vi "Motor_Excel_to_Array(OK).vi"() -> ()   [LabVIEW 2016]
uses:
  <vilib>/addons/_office/excel.llb/Excel Get Data ([dbl]).vi
  <vilib>/Utility/NIReport.llb/NI_report.lvclass
  <vilib>/Utility/NIReport.llb/Excel/NI_Excel.lvclass
  <vilib>/addons/_office/NI_ReportGenerationToolkit.lvlib
  <vilib>/gmath/NI_Gmath.lvlib
panel:
  in  "Path":path=path "C:/Users/YENPEI/Desktop/LabView/20.2_Motor_Performace - accel/Peak.xls"
  in  "Tab Control":T1(tab)
  out "XY Graph":cluster{"data":dbl[], "data":dbl[]}[](graph)
  out "Speed -MotorTorque - Curve":T2(graph)={"array type (2D Dbl)"=[0.0, 5.0, 10.0, 15.0, 20.0, 25.0, 30.0, 35.0, 40.0, 45.0, 50.0, 55.0, 60.0, 65.0, 70.0, 75.0, 80.0, 85.0, 90.0, 95.0, 100.0, 105.0, 110.0, 115.0, 120.0, 125.0, 130.0, 135.0, 140.0, 145.0, 150.0, 155.0, 160.0, 165.0, 170.0, 175.0, 180.0, 185.0, 190.0, 195.0, 200.0, 205.0, 210.0, 215.0, 220.0, 225.0, 230.0, 235.0, 240.0, 245.0], "array type (2D Dbl)"=[7.64, 4.95, 6.83, 9.7, 4.25, 5.21, 3.69, 9.63, 7.28, 4.87, 6.61, 3.48, 3.51, 5.43, 7.79, 2.74, 3.77, 9.97, 2.54, 5.19, 9.7, 5.12, 1.95, 1.46, 2.93, 2.02, 4.5, 5.86, 6.09, 5.11, 1.22, 8.82, 1.81, 7.21, 5.19, 4.2, 7.97, 6.75, 2.71, 3.86, 1.49, 3.44, 5.75, 5.05, 3.16, 8.68, 8.7, 4.07, 5.28, 3.4]}
  out "Motor Max Torque":T2(graph)={"array type (2D Dbl)"=[0.0, 5.0, 10.0, 15.0, 20.0, 25.0, 30.0, 35.0, 40.0, 45.0, 50.0, 55.0, 60.0, 65.0, 70.0, 75.0, 80.0, 85.0, 90.0, 95.0, 100.0, 105.0, 110.0, 115.0, 120.0, 125.0, 130.0, 135.0, 140.0, 145.0, 150.0, 155.0, 160.0, 165.0, 170.0, 175.0, 180.0, 185.0, 190.0, 195.0, 200.0, 205.0, 210.0, 215.0, 220.0, 225.0, 230.0, 235.0, 240.0, 245.0], "array type (2D Dbl)"=[7.64, 4.95, 6.83, 9.7, 4.25, 5.21, 3.69, 9.63, 7.28, 4.87, 6.61, 3.48, 3.51, 5.43, 7.79, 2.74, 3.77, 9.97, 2.54, 5.19, 9.7, 5.12, 1.95, 1.46, 2.93, 2.02, 4.5, 5.86, 6.09, 5.11, 1.22, 8.82, 1.81, 7.21, 5.19, 4.2, 7.97, 6.75, 2.71, 3.86, 1.49, 3.44, 5.75, 5.05, 3.16, 8.68, 8.7, 4.07, 5.28, 3.4]}
  out "Motor Power Curve":T2(graph)={"array type (2D Dbl)"=[0.0, 5.0, 10.0, 15.0, 20.0, 25.0, 30.0, 35.0, 40.0, 45.0, 50.0, 55.0, 60.0, 65.0, 70.0, 75.0, 80.0, 85.0, 90.0, 95.0, 100.0, 105.0, 110.0, 115.0, 120.0, 125.0, 130.0, 135.0, 140.0, 145.0, 150.0, 155.0, 160.0, 165.0, 170.0, 175.0, 180.0, 185.0, 190.0, 195.0, 200.0, 205.0, 210.0, 215.0, 220.0, 225.0, 230.0, 235.0, 240.0, 245.0], "array type (2D Dbl)"=[7.64, 4.95, 6.83, 9.7, 4.25, 5.21, 3.69, 9.63, 7.28, 4.87, 6.61, 3.48, 3.51, 5.43, 7.79, 2.74, 3.77, 9.97, 2.54, 5.19, 9.7, 5.12, 1.95, 1.46, 2.93, 2.02, 4.5, 5.86, 6.09, 5.11, 1.22, 8.82, 1.81, 7.21, 5.19, 4.2, 7.97, 6.75, 2.71, 3.86, 1.49, 3.44, 5.75, 5.05, 3.16, 8.68, 8.7, 4.07, 5.28, 3.4]}
  out "Speed - RoadTorque - Curve2":T2(graph)={"array type (2D Dbl)"=[0.0, 5.0, 10.0, 15.0, 20.0, 25.0, 30.0, 35.0, 40.0, 45.0, 50.0, 55.0, 60.0, 65.0, 70.0, 75.0, 80.0, 85.0, 90.0, 95.0, 100.0, 105.0, 110.0, 115.0, 120.0, 125.0, 130.0, 135.0, 140.0, 145.0, 150.0, 155.0, 160.0, 165.0, 170.0, 175.0, 180.0, 185.0, 190.0, 195.0, 200.0, 205.0, 210.0, 215.0, 220.0, 225.0, 230.0, 235.0, 240.0, 245.0], "array type (2D Dbl)"=[7.64, 4.95, 6.83, 9.7, 4.25, 5.21, 3.69, 9.63, 7.28, 4.87, 6.61, 3.48, 3.51, 5.43, 7.79, 2.74, 3.77, 9.97, 2.54, 5.19, 9.7, 5.12, 1.95, 1.46, 2.93, 2.02, 4.5, 5.86, 6.09, 5.11, 1.22, 8.82, 1.81, 7.21, 5.19, 4.2, 7.97, 6.75, 2.71, 3.86, 1.49, 3.44, 5.75, 5.05, 3.16, 8.68, 8.7, 4.07, 5.28, 3.4]}
  out "XY Graph 2":cluster{"data":dbl[], "data":dbl[]}[](graph)
  out "slope_value_(%) 2":dbl format="%.1f"
  out "Motor_Max_Torque(Nm) 2":dbl format="%.2f"
  out "Motor_Max_Power(kW)":dbl format="%.2f"
  out "Vehicle_speed_Hi(kph)@ Slope":dbl format="%.2f"
  out "Vehicle_speed_Lo(kph)@ Slope":dbl format="%.2f"
  out "Tire_Torque Array(kph_Nm)":dbl[][](array[numeric]) format="%#.1f"
  out "Motor_Torque_Orignal":dbl[][](array[numeric])
  in  "window state (normal)":T3(ring)=enum."normal"
  in  "report type":T4(ring)=enum."Excel"
  out "Vehicle_speed_(m/s)":dbl[](array[numeric])
  out "Vehicle_speed_(km/h)":dbl[](array[numeric])
  out "Road_Resistance_Array (kph_Nm)":dbl[][](array[numeric]) format="%#.1f"
  out "Road_Load 1 (Aero)":dbl[](array[numeric])
  out "Road_Load 2 (Roll)":dbl=0.7
  out "Road_Load_3(slope)":dbl=0.7
  out "New_Motor_Torque_Array (rpm_Nm)":dbl[][](array[numeric])
  in  "Road_Slope_(%)":sgl(slide) min=0 max=30 step=1 scale=0.0..30.0
  in  "Trie_HWRatio_(%)":dbl=75.0
  out "Front_Area(m^2)":dbl
  out "Tire_Radius(m)":dbl=0.3835
  in  "Mass_AddFactor_(-)":dbl=1.04
  in  "Tire_Diameter_ (in)":dbl=17.5
  in  "Tire_Height_(mm)":dbl=215.0
  out "Trie Skip coefficient(-)":dbl=0.03
  in  "Reducer_Ratio_(-)":dbl=5.13
  out "rolling friction_coefficient_(-)":dbl=0.01
  out "Airdensity(kg/m^3)":dbl=1.225
  out "Graviational_constant_(m/s^2)":dbl=9.81
  out "areo_dynamic_coefficient_(-)":dbl=0.7
  in  "Powertrain_eff_(%)":dbl=85.0
  in  "Vehicle_Load_(kg)":dbl=9900.0
  in  "Vehicle_width_(m)":dbl=2.3
  in  "Vehicle_Height_m)":dbl=3.0
  in  "Front_Area_constant(-)":dbl=1.0
  out "slope_value_(%)":dbl format="%.1f"
  in  "Table":bool=TRUE
  out "Max slope_angle_(deg)":dbl format="%.1f"
  out "Max slope_value_(%)":dbl format="%.1f"
  out "Vehicle_Max_speed_(kph)":dbl format="%.2f"
  in  "Torque _(Nm) @ Max_Motor_speed":dbl=500.0
  in  "Max_Motor_speed (rpm)":dbl=4000.0
  out "Vehicle_Max_speed":dbl format="%.2f"
  out "Road_Loading_Torque":dbl format="%.2f"
  out "Vehicle_Torque_Max_speed":dbl format="%.2f"
  out "Motor_Max_Torque(Nm)":dbl format="%.2f"
  in  "Motor _Max Torque (Nm)":dbl=2000.0
  in  "Motor_speed @ Max Torque (rpm)":dbl=1000.0
  out "Vehicle_spped_Array (m/s_Nm) 2":dbl[][](array[numeric])
  out "Vehicle_Total_Array":dbl[][](array[numeric]) format="%.2f"
  out "vehicle speed vs Distance":cluster{dbl[], dbl[]}(graph)
  out "Aceel time vs vehicle speed":cluster{dbl[], dbl[]}(graph)
  in  "Max Distance [m]":i32=400 min=0 max=400 step=1
  in  "Max Accel  time [sec]":i32=20 min=0 max=20 step=1
  in  "Max Items":i32=29 min=0 max=30 step=1
  in  "Stop Mode":i32 min=0 max=3 step=1
  in  "Max Vehicel Speed [kph]":i32=60 min=0 max=100 step=1
  out "Aceel time vs Distance":cluster{dbl[], dbl[]}(graph)
  out "Accel_Result":dbl[](array[numeric]) format="%.2f"
  # "Max Vehicle Speed\nBetween"
  # "~"
  # "最大爬坡度"
  # "極速(km/hr)"
  # "檢查馬達最大轉速 Nmax (rpm)     與扭力(Nm)"
  # "¦pªGTable data µL°¨¹F³Ì¤jÂà³t , Table¶s Disable¡A«h¤â°Ê¿é¤J¤U¤è"
  # "檢查馬達最大扭力(Nm)"
  # "¦pªGTable data µL°¨¹F³Ì¤j§á¤O ,  Table¶s Disable ¡A«h¤â°Ê¿é¤J¤U¤è"
  # "Finak \n車速 m/s"
  # "Motor\nrpm"
  # "Motor\nrpm"
  # "Tire Drive\nN"
  # "Aceel Drive\nN"
  # "Aceel \n1/sec"
  # "time  \nsec"
  # "車速 m/s"
  # "車速 kph"
  # "Drag"
  # "Roll"
  # "Drag+Roll"
  # "Distance\nm"
  # "Final \n車速 kph"
  # "Total Time\n[sec]"
  # "Total Distance\n[m]"
  # "Mode =0"
  # "Max =30"
  # "Item"
  # "Final \n車速 kph"
  # "Total Time\n[sec]"
  # "Total Distance\n[m]"
  # "Mode =1"
  # "Max =100"
  # "Mode =2"
  # "Max =15"
  # "Mode =3"
  # "Max =300"
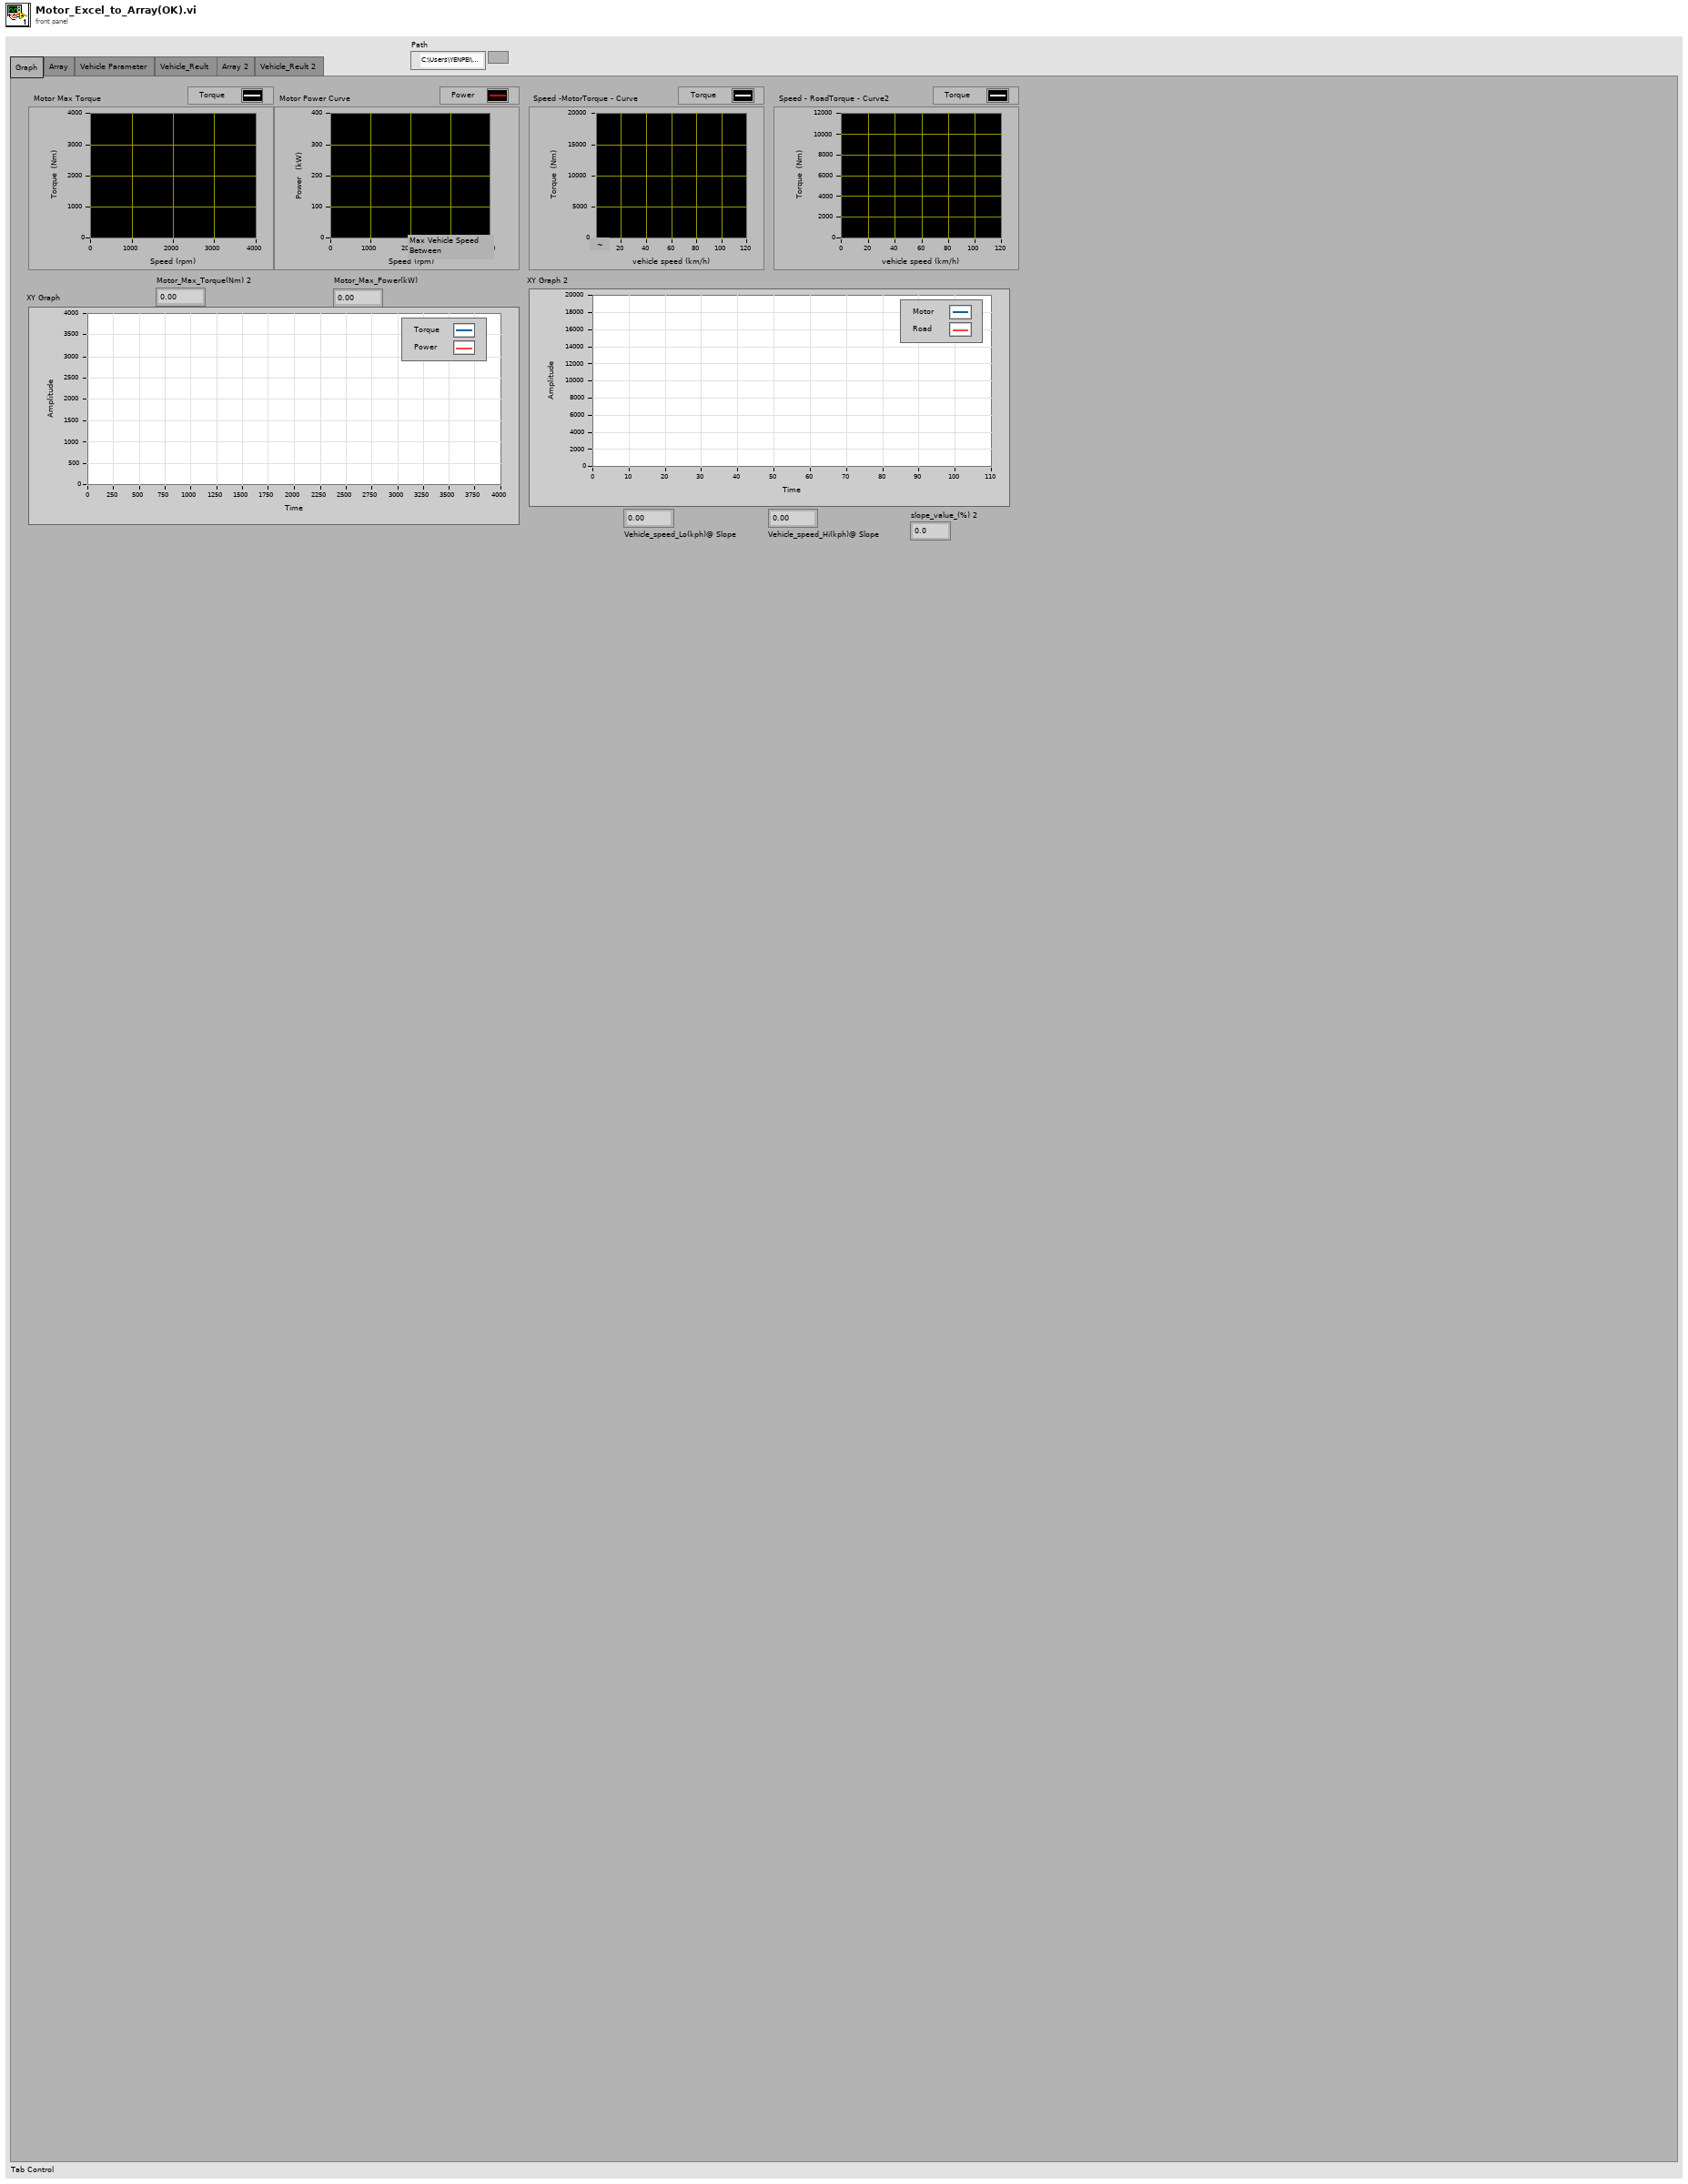
[diagram p1: front panel]
types:
  T1 = enum32{"Graph", "Array", "Vehicle Parameter", "Vehicle_Reult", "Array 2", "Vehicle_Reult 2"}
  T2 = cluster{"array type (2D Dbl)":dbl[], "array type (2D Dbl)":dbl[]}
  T3 = enum16{"maximized", "minimized", "normal", "no change"}
  T4 = enum16{"Standard Report", "HTML", "Word", "Excel"}
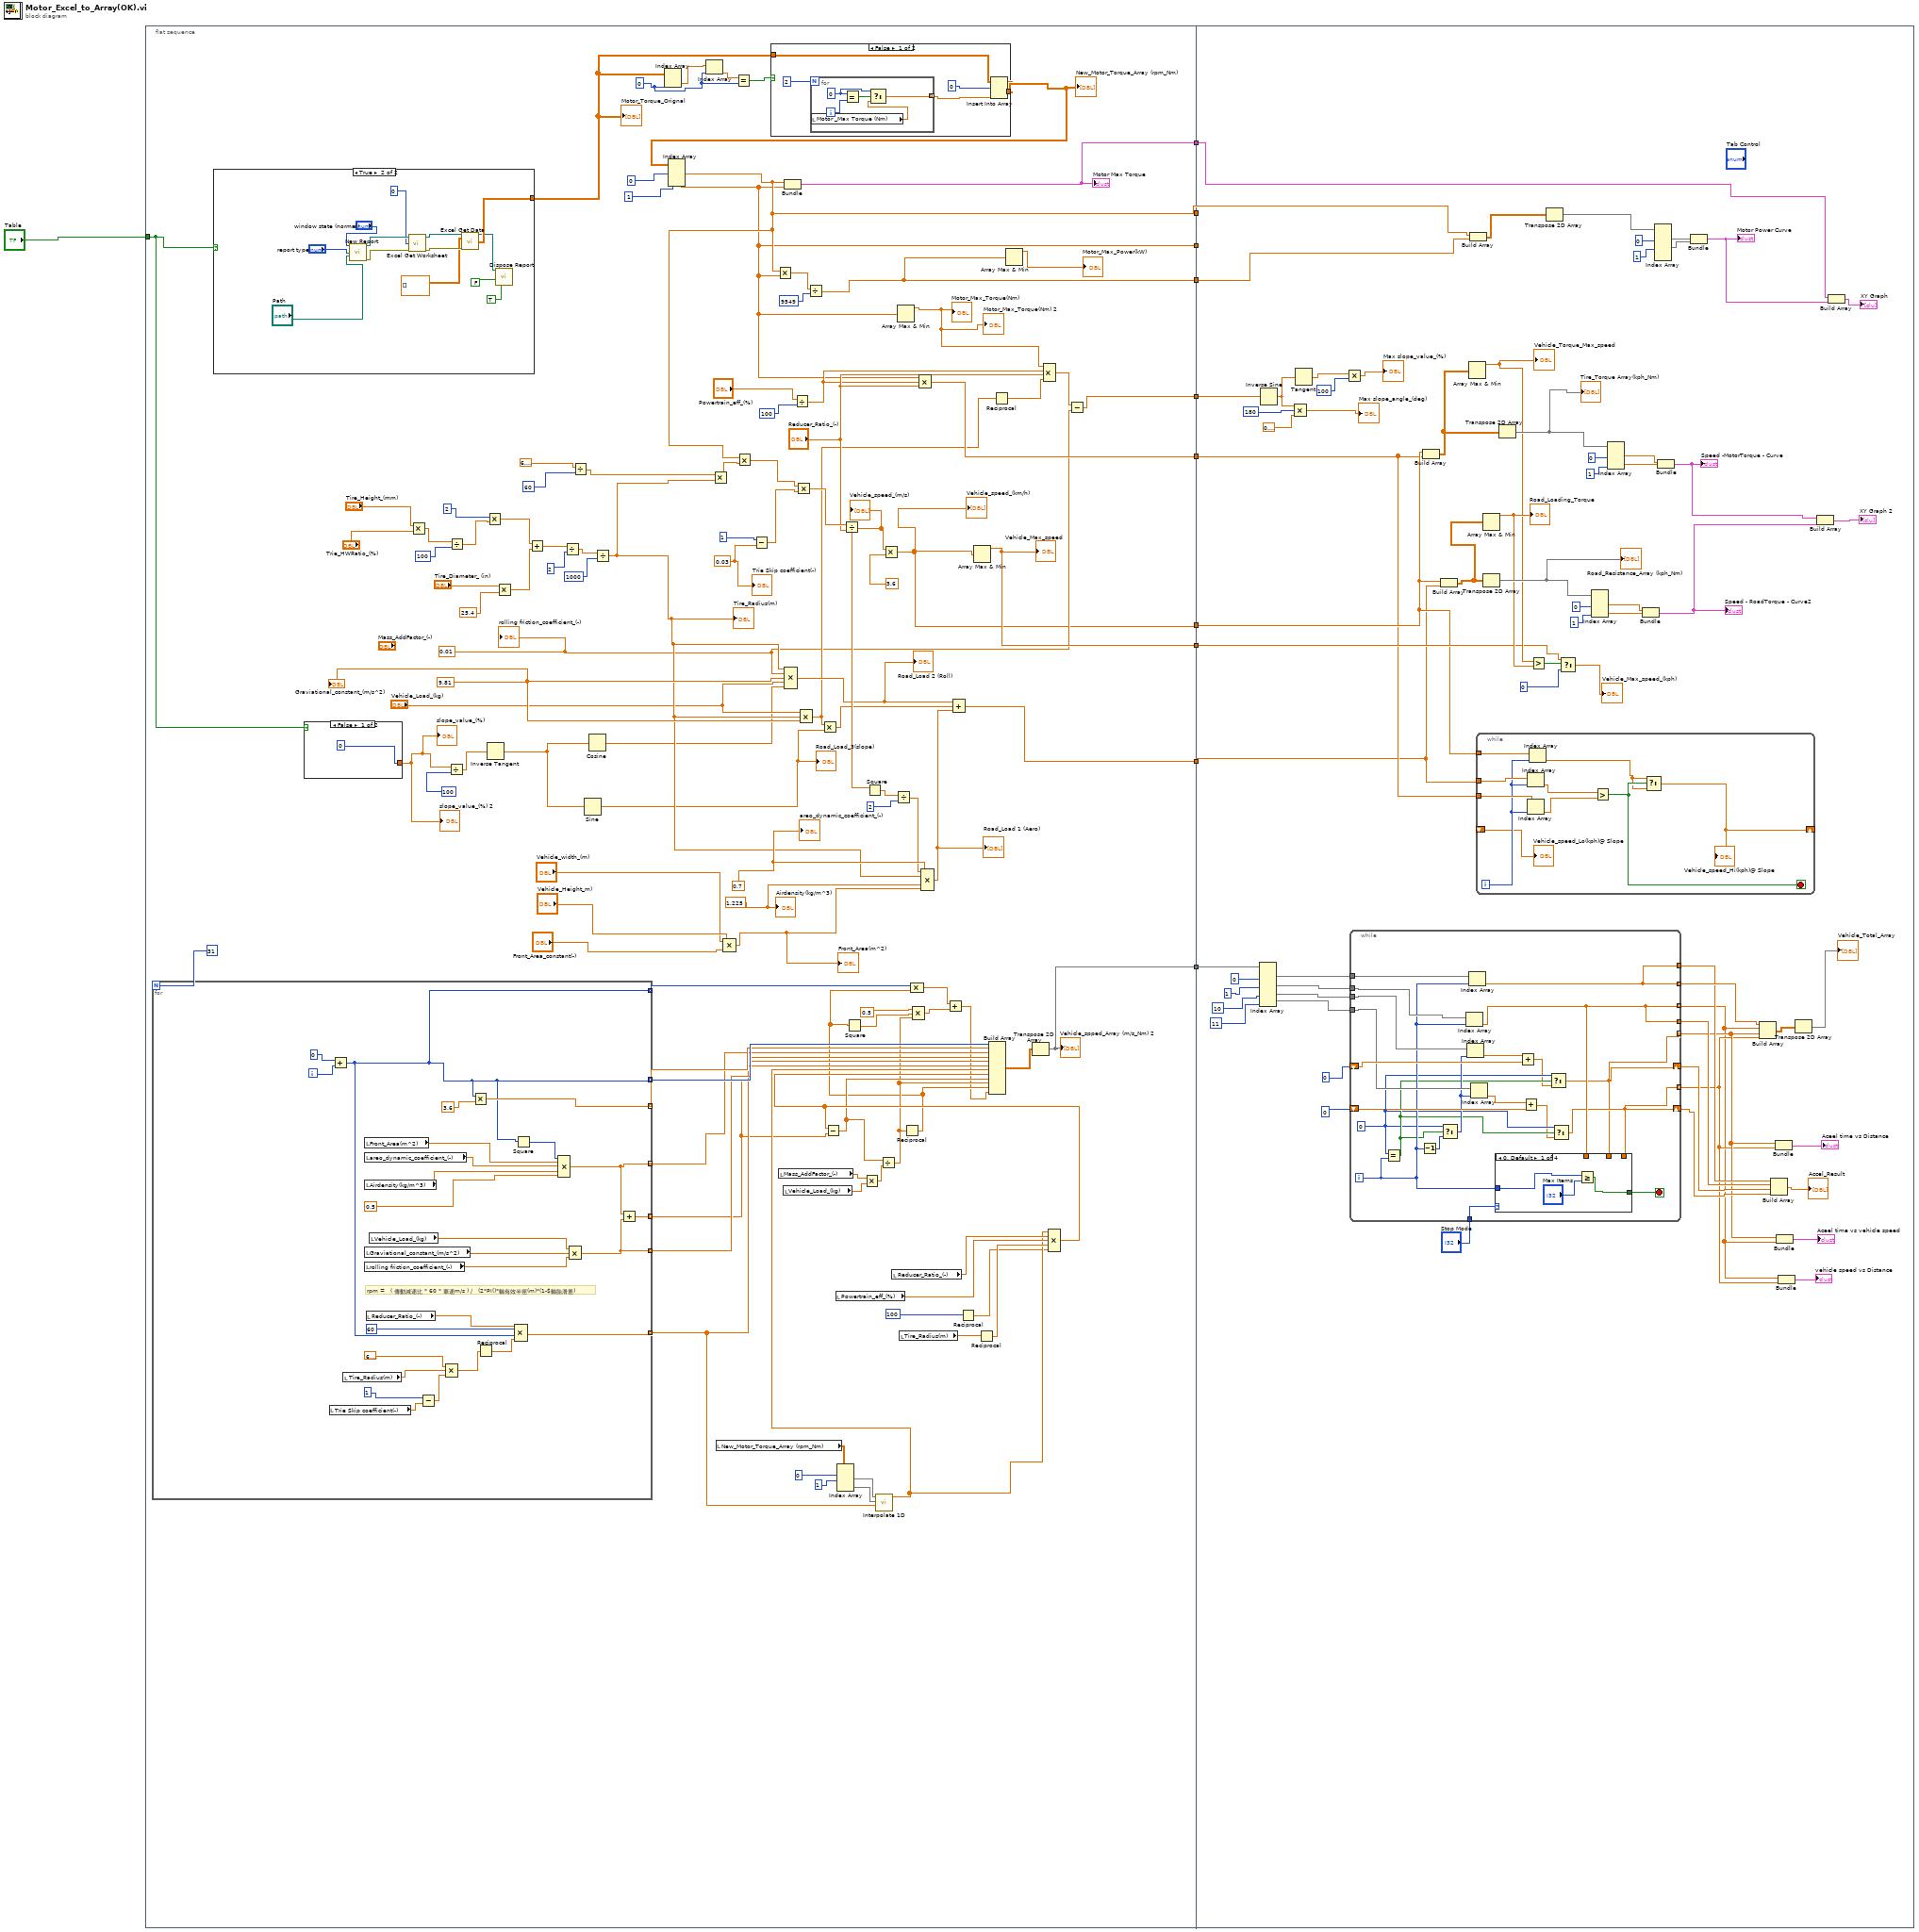
[diagram p0: block diagram]
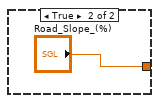
[diagram p3: hidden frame]
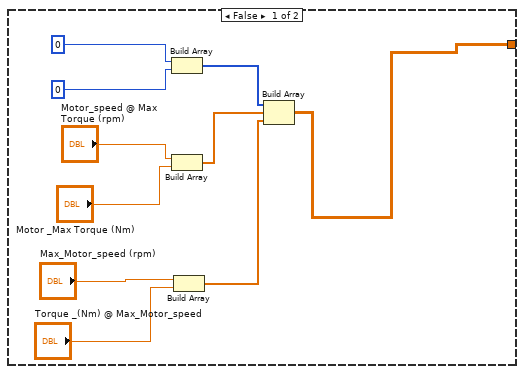
[diagram p4: hidden frame]
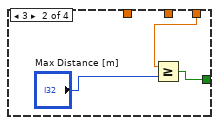
[diagram p5: hidden frame]
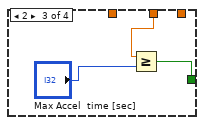
[diagram p6: hidden frame]
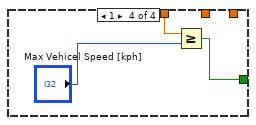
[diagram p7: hidden frame]
diagram:
  n1 = flat-sequence {
    tunnel: [w22] -> w10
    tunnel: [w15] -> w9
    tunnel: [w23] -> w8
    tunnel: [w60] -> w7
    tunnel: [w83] -> w6
    tunnel: [w82] -> w5
    tunnel: "Table" -> [w72]
    tunnel: [w71] -> w4
    tunnel: [w63] -> w3
    tunnel: [w59] -> w2
    tunnel: [w24] -> w1
    tunnel: w10 -> [_]
    tunnel: w9 -> [w245]
    tunnel: w8 -> [w246]
    tunnel: w7 -> [w186]
    tunnel: w6 -> [w185]
    tunnel: w5 -> [w184]
    tunnel: w4 -> [w227]
    tunnel: w3 -> [w219]
    tunnel: w2 -> [w218]
    tunnel: w1 -> [w212]
    frame #0 {
      w19 = 0
      w90 = 0.7
      w64 = 0.01
      w89 = 1.225
      w79 = 9.81
      w98 = 0.03
      n2 = for {
        N: 31 -> [_]
        tunnel: [w133] -> w56 mode=indexing
        tunnel: [w155] -> w55 mode=indexing
        tunnel: [w146] -> w54 mode=indexing
        tunnel: [w145] -> w53 mode=indexing
        tunnel: [w144] -> w38 mode=indexing
        tunnel: [w134] -> w48 mode=indexing
        tunnel: [w133] -> w33 mode=indexing
        i -> [w157]
        # "rpm =   ( 傳動減速比 * 60 * 車速m/s ) /   (2*PI()*輪有效半徑(m)*(1-$輪胎滑差)"
        n3 = local read "Trie Skip coefficient(-)"() -> (w137:dbl)
        n4 = Add(x=0, y=w157) -> (x+y=w133:i32)
        n5 = local read "Tire_Radius(m)"() -> (w135:dbl)
        n6 = local read "Front_Area(m^2)"() -> (w148:dbl)
        n7 = local read "areo_dynamic_coefficient_(-)"() -> (w149:dbl)
        n8 = local read "Airdensity(kg/m^3)"() -> (w150:dbl)
        n9 = local read "Graviational_constant_(m/s^2)"() -> (w152:dbl)
        n10 = local read "rolling friction_coefficient_(-)"() -> (w153:dbl)
        n11 = local read "Reducer_Ratio_(-)"() -> (w143:dbl)
        n12 = local read "Vehicle_Load_(kg)"() -> (w154:dbl)
        n13 = Subtract(x=1, y=w137) -> (x-y=w136:dbl)
        n14 = Compound Arithmetic op=MULTIPLY(6.283185307179586, w135, w136) -> (w140:dbl)
        n15 = Multiply(x=w133, y=3.6) -> (x*y=w155:dbl)
        n16 = Reciprocal(x=w140) -> (1/x=w141:dbl)
        n17 = Compound Arithmetic op=MULTIPLY(w143, 60, w133, w141) -> (w134:dbl)
        n18 = Square(x=w133) -> (x^2=w147:i32)
        n19 = Compound Arithmetic op=MULTIPLY(w147, w148, w149, w150, 0.5) -> (w146:dbl)
        n20 = Compound Arithmetic op=MULTIPLY(w154, w152, w153) -> (w145:dbl)
        n21 = Add(x=w146, y=w145) -> (x+y=w144:dbl)
      }
      n22 = case shown="True" w72 {
        tunnel: [w165 w177] -> w17
        frame False {
          n23 = Build Array(0, 0) -> (w166:i32[])
          n24 = Build Array("Motor_speed @ Max Torque (rpm)", "Motor _Max Torque (Nm)") -> (w161:dbl[])
          n25 = Build Array("Max_Motor_speed (rpm)", "Torque _(Nm) @ Max_Motor_speed") -> (w164:dbl[])
          n26 = Build Array(w166, w161, w164) -> (w165:dbl[][])
        }
        frame True {
          n27 = call <vilib>:"New Report.vi"("window state (normal)"="window state (normal)", "report type"="report type", "template (empty)"="Path") -> ("report out"=w182:refnum<class "NI_report.lvclass">, "error out"=w183:errorcluster)  [unwired: 11 in]
          n28 = call <vilib>:"Excel Get Worksheet.vi"("report in"=w182, "worksheet index (0)"=0, "error in (no error)"=w183) -> ("report out"=w181:refnum<class "NI_report.lvclass">, "error out"=w180:errorcluster)  [unwired: 11 in]
          n29 = call-poly <vilib>:"Excel Get Data.vi"("report in"=w181, "data type"=dbl[][] [], "error in (no error)"=w180) -> ("report out"=w173:refnum<class "NI_report.lvclass">, "data"=w177:dbl[][])  [unwired: 10 in, 1 out]
          n30 = call-dynamic "Dispose Report.vi"("report in"=w173, "save changes? (F)"=FALSE, "close report? (T)"=TRUE) -> ()  [unwired: 12 in, 1 out]
        }
      }
      "Motor_Torque_Orignal" <- w17
      n31 = case shown="False" w72 {
        tunnel: [0 "Road_Slope_(%)"] -> w12
        frame False {
        }
        frame True {
        }
      }
      "slope_value_(%)" <- w12
      "slope_value_(%) 2" <- w12
      n32 = Multiply(x="Tire_Height_(mm)", y="Trie_HWRatio_(%)") -> (x*y=w112:dbl)
      n33 = Divide(x=w12, y=100) -> (x/y=w75:sgl)
      n34 = Divide(x=w112, y=100) -> (x/y=w107:dbl)
      n35 = Multiply(x=2, y=w107) -> (x*y=w106:dbl)
      n36 = Inverse Tangent(1:w75) -> (0:w76:sgl)
      n37 = Multiply(x="Tire_Diameter_ (in)", y=25.4) -> (x*y=w105:dbl)
      n38 = Add(x=w106, y=w105) -> (x+y=w102:dbl)
      n39 = Divide(x=w102, y=2) -> (x/y=w100:dbl)
      n40 = Divide(x=6.283185307179586, y=60) -> (x/y=w115:dbl)
      n41 = Sine(x=w76) -> (sin(x)=w58:sgl)
      "Road_Load_3(slope)" <- w58
      n42 = Cosine(x=w76) -> (cos(x)=w68:sgl)
      n43 = Divide(x=w100, y=1000) -> (x/y=w77:dbl)
      "Tire_Radius(m)" <- w77
      n44 = Index Array(array=w17, index (row)=w19) -> (element=w21:dbl[])  [unwired: 1 in]
      n45 = Index Array(array=w21, index=w19) -> (element=w20:dbl)
      n46 = Multiply(x=w115, y=w77) -> (x*y=w104:dbl)
      n47 = local read "New_Motor_Torque_Array (rpm_Nm)"() -> (w47:dbl[][])
      n48 = Compound Arithmetic op=MULTIPLY("Vehicle_width_(m)", "Vehicle_Height_m)", "Front_Area_constant(-)") -> (w85:dbl)
      "Front_Area(m^2)" <- w85
      n49 = Equal?(x=w20, y=w19) -> (x = y?=w18:bool)
      n50 = Subtract(x=1, y=w98) -> (x-y=w97:dbl)
      n51 = case shown="False" w18 {
        tunnel: [w126 w132] -> w13
        tunnel: w17 -> [w122 w132]
        frame False {
          n52 = for {
            N: 2 -> [_]
            tunnel: [w128] -> w124 mode=indexing
            i -> [w131]
            w129 = 0
            n53 = local read "Motor _Max Torque (Nm)"() -> (w127:dbl)
            n54 = Equal?(x=w129, y=w131) -> (x = y?=w130:bool)
            n55 = Select(t=w129, s=w130, f=w127) -> (s? t:f=w128:dbl)
          }
          n56 = Insert Into Array(array=w122, index (row)=0, new element=w124) -> (w126:dbl[][])  [unwired: 1 in]
        }
        frame True {
        }
      }
      "New_Motor_Torque_Array (rpm_Nm)" <- w13
      n57 = Index Array "Index Array"(array=w13, index (col) #1=0 ("disabled index (col)"), index (col) #2=1 ("index (col)")) -> (element #1=w23:dbl[], element #2=w22:dbl[])  [unwired: 2 in]
      n58 = Multiply(x=w23, y=w104) -> (x*y=w96:dbl[])
      n59 = Multiply(x=w23, y=w22) -> (x*y=w118:dbl[])
      n60 = local read "Mass_AddFactor_(-)"() -> (w37:dbl)
      n61 = local read "Vehicle_Load_(kg)"() -> (w36:dbl)
      n62 = Bundle "Bundle"("data"=w23, "data"=w22) -> (w59:cluster{"data":dbl[], "data":dbl[]})  [unwired: 1 in]
      "Motor Max Torque" <- w59
      n63 = Compound Arithmetic op=MULTIPLY(w77, w64, w79, "Vehicle_Load_(kg)", w68) -> (w80:dbl)
      "Road_Load 2 (Roll)" <- w80
      n64 = Divide(x="Powertrain_eff_(%)", y=100) -> (x/y=w61:dbl)
      n65 = Multiply(x=w96, y=w97) -> (x*y=w95:dbl[])
      n66 = Compound Arithmetic op=MULTIPLY("Vehicle_Load_(kg)", w77, w79) -> (w66:dbl)
      n67 = Divide(x=w118, y=9549) -> (x/y=w15:dbl[])
      n68 = Multiply(x=w66, y=w58) -> (x*y=w67:dbl)
      n69 = local read "Powertrain_eff_(%)"() -> (w50:dbl)
      n70 = Index Array(array=w47, index (col) #1=1, index (col) #2=0) -> (element #1=w44:dbl[], element #2=w43:dbl[])  [unwired: 2 in]
      n71 = Divide(x=w95, y="Reducer_Ratio_(-)") -> (x/y=w93:dbl[])
      "Vehicle_speed_(m/s)" <- w93
      n72 = Multiply(x=w37, y=w36) -> (x*y=w35:dbl)
      n73 = Square(x=w93) -> (x^2=w91:dbl[])
      n74 = call <vilib>:"Interpolate 1D.vi"("xi"=w48, "X"=w43, "Y"=w44) -> ("yi"=w42:dbl[])  [unwired: 6 in, 2 out]
      n75 = Multiply(x=w93, y=3.6) -> (x*y=w60:dbl[])
      "Vehicle_speed_(km/h)" <- w60
      n76 = local read "Reducer_Ratio_(-)"() -> (w52:dbl)
      n77 = Divide(x=w91, y=2) -> (x/y=w78:dbl[])
      n78 = Array Max & Min(array=w22) -> (max value=w16:dbl)  [unwired: 3 out]
      "Motor_Max_Torque(Nm)" <- w16
      "Motor_Max_Torque(Nm) 2" <- w16
      n79 = local read "Tire_Radius(m)"() -> (w51:dbl)
      n80 = Compound Arithmetic op=MULTIPLY(w22, w61, "Reducer_Ratio_(-)") -> (w83:dbl[])
      n81 = Compound Arithmetic op=MULTIPLY(w78, w77, w90, w89, w85) -> (w81:dbl[])
      "Road_Load 1 (Aero)" <- w81
      n82 = Compound Arithmetic op=ADD(w80, w67, w81) -> (w82:dbl[])
      n83 = Reciprocal(x=100) -> (1/x=w40:dbl)
      n84 = Array Max & Min(array=w60) -> (max value=w71:dbl)  [unwired: 3 out]
      "Vehicle_Max_speed" <- w71
      n85 = Reciprocal(x=w51) -> (1/x=w49:dbl)
      n86 = Reciprocal(x=w66) -> (1/x=w65:dbl)
      n87 = Array Max & Min(array=w15) -> (max value=→"Motor_Max_Power(kW)":dbl)  [unwired: 3 out]
      n88 = Compound Arithmetic op=MULTIPLY(w16, w61, "Reducer_Ratio_(-)", w65) -> (w62:dbl)
      n89 = Compound Arithmetic op=MULTIPLY(w42, w52, w50, w49, w40) -> (w39:dbl[])
      n90 = Subtract(x=w39, y=w38) -> (x-y=w34:dbl[])
      n91 = Divide(x=w34, y=w35) -> (x/y=w30:dbl[])
      n92 = Reciprocal(x=w30) -> (1/x=w29:dbl[])
      n93 = Square(x=w29) -> (x^2=w31:dbl[])
      n94 = Compound Arithmetic op=MULTIPLY(w33, w29) -> (w28:dbl[])
      n95 = Compound Arithmetic op=MULTIPLY(0.5, w31, w30) -> (w27:dbl[])
      n96 = Add(x=w28, y=w27) -> (x+y=w26:dbl[])
      n97 = Build Array(w56, w55, w54, w53, w38, w48, w42, w39, w34, w30, w29, w26) -> (w25:dbl[][])
      n98 = Transpose 2D Array(2D array=w25) -> (transposed array=w24:dbl[][])
      "Vehicle_spped_Array (m/s_Nm) 2" <- w24
      n99 = Subtract(x=w62, y=w64) -> (x-y=w63:dbl)
      "Trie Skip coefficient(-)" <- w98
      "Graviational_constant_(m/s^2)" <- w79
      "Airdensity(kg/m^3)" <- w89
      "rolling friction_coefficient_(-)" <- w64
      "areo_dynamic_coefficient_(-)" <- w90
    }
    frame #1 {
      n100 = Index Array(array=w212, index (col) #1=0 ("disabled index (col)"), index (col) #2=1 ("index (col)"), index (col) #3=10, index (col) #4=11) -> (element #1=w207:dbl[], element #2=w206:dbl[], element #3=w205:dbl[], element #4=w204:dbl[])  [unwired: 4 in]
      n101 = Inverse Sine(1:w219) -> (0:w224:dbl)
      n102 = Compound Arithmetic op=MULTIPLY(w224, 180, 0.3183098861837907) -> (→"Max slope_angle_(deg)":dbl)
      n103 = Tangent(1:w224) -> (0:w222:dbl)
      n104 = Multiply(x=w222, y=100) -> (x*y=→"Max slope_value_(%)":dbl)
      n105 = while {
        tunnel: w207 -> [w280]
        tunnel: w206 -> [w279]
        tunnel: w205 -> [w278]
        tunnel: w204 -> [w277]
        shift-right: [w264] -> w194
        shift-left: 0 -> [w282]
        shift-right: [w265] -> w196
        shift-left: 0 -> [w283]
        tunnel: [w273] -> w201 mode=indexing
        tunnel: [w272] -> w187 mode=indexing
        tunnel: [w264] -> w190 mode=indexing
        tunnel: [w265] -> w189 mode=indexing
        tunnel: "Stop Mode" -> [w274]
        tunnel: [w273] -> w193
        tunnel: [w272] -> w192
        i -> [w270]
        stop <- w281 stop-if-true
        w267 = 0
        n106 = Equal?(x=w267, y=w270) -> (x = y?=w268:bool)
        n107 = Decrement(x=w270) -> (x-1=w271:i32)
        n108 = Select(t=w267, s=w268, f=w271) -> (s? t:f=w269:i32)
        n109 = Index Array(array=w279, index=w270) -> (element=w272:dbl)
        n110 = Index Array(array=w278, index=w269) -> (element=w276:dbl)
        n111 = Index Array(array=w280, index=w270) -> (element=w273:dbl)
        n112 = Index Array(array=w277, index=w269) -> (element=w275:dbl)
        n113 = Add(x=w276, y=w282) -> (x+y=w263:dbl)
        n114 = Add(x=w275, y=w283) -> (x+y=w266:dbl)
        n115 = Select(t=w267, s=w268, f=w263) -> (s? t:f=w264:dbl)
        n116 = Select(t=w267, s=w268, f=w266) -> (s? t:f=w265:dbl)
        n117 = case shown="0, Default" w274 {
          tunnel: [w285 w287 w290 w294] -> w281
          tunnel: w270 -> [w286 _ _ _]
          tunnel: w272 -> [_ _ _ w293]
          tunnel: w264 -> [_ _ w291 _]
          tunnel: w265 -> [_ w288 _ _]
          frame 0, Default {
            n118 = Greater Or Equal?(x=w286, y="Max Items") -> (x >= y?=w285:bool)
          }
          frame 3 {
            n119 = Greater Or Equal?(x=w288, y="Max Distance [m]") -> (x >= y?=w287:bool)
          }
          frame 2 {
            n120 = Greater Or Equal?(x=w291, y="Max Accel  time [sec]") -> (x >= y?=w290:bool)
          }
          frame 1 {
            n121 = Greater Or Equal?(x=w293, y="Max Vehicel Speed [kph]") -> (x >= y?=w294:bool)
          }
        }
      }
      n122 = Build Array(w186, w185) -> (w233:dbl[][])
      n123 = Build Array(w186, w184) -> (w234:dbl[][])
      n124 = Array Max & Min(array=w233) -> (max value=w230:dbl)  [unwired: 3 out]
      "Vehicle_Torque_Max_speed" <- w230
      n125 = Build Array(w246, w245) -> (w247:dbl[][])
      n126 = while {
        tunnel: w186 -> [w262]
        tunnel: w185 -> [w261]
        tunnel: w184 -> [w260]
        shift-right: [w256] -> _
        shift-left: _ -> [w254]
        i -> [w259]
        stop <- w255 stop-if-true
        n127 = Index Array(array=w260, index=w259) -> (element=w258:dbl)
        n128 = Index Array(array=w261, index=w259) -> (element=w257:dbl)
        n129 = Index Array(array=w262, index=w259) -> (element=w253:dbl)
        n130 = Greater?(x=w258, y=w257) -> (0:w255:bool)
        n131 = Select(t=w253, s=w255, f=w253) -> (s? t:f=w256:dbl)
        "Vehicle_speed_Hi(kph)@ Slope" <- w256
        "Vehicle_speed_Lo(kph)@ Slope" <- w254
      }
      n132 = Array Max & Min(array=w234) -> (max value=w231:dbl)  [unwired: 3 out]
      "Road_Loading_Torque" <- w231
      n133 = Transpose 2D Array(2D array=w234) -> (transposed array=w235:dbl[][])
      "Road_Resistance_Array (kph_Nm)" <- w235
      n134 = Transpose 2D Array(2D array=w233) -> (transposed array=w240:dbl[][])
      "Tire_Torque Array(kph_Nm)" <- w240
      n135 = Greater?(x=w230, y=w231) -> (0:w229:bool)
      n136 = Transpose 2D Array(2D array=w247) -> (transposed array=w252:dbl[][])
      n137 = Select(t=w227, s=w229, f=0 ("disabled index (col)")) -> (s? t:f=→"Vehicle_Max_speed_(kph)":dbl)
      n138 = Index Array "Index Array"(array=w235, index (col) #1=0 ("disabled index (col)"), index (col) #2=1 ("index (col)")) -> (element #1=w237:dbl[], element #2=w236:dbl[])  [unwired: 2 in]
      n139 = Index Array "Index Array"(array=w240, index (col) #1=0 ("disabled index (col)"), index (col) #2=1 ("index (col)")) -> (element #1=w242:dbl[], element #2=w241:dbl[])  [unwired: 2 in]
      n140 = Bundle "Bundle"(w237, w236) -> (w214:cluster{dbl[], dbl[]})  [unwired: 1 in]
      "Speed - RoadTorque - Curve2" <- w214
      n141 = Index Array "Index Array"(array=w252, index (col) #1=0 ("disabled index (col)"), index (col) #2=1 ("index (col)")) -> (element #1=w249:dbl[], element #2=w248:dbl[])  [unwired: 4 in, 1 out]
      n142 = Bundle "Bundle"(w242, w241) -> (w215:cluster{dbl[], dbl[]})  [unwired: 1 in]
      "Speed -MotorTorque - Curve" <- w215
      n143 = Bundle "Bundle"(w249, w248) -> (w216:cluster{dbl[], dbl[]})  [unwired: 1 in]
      "Motor Power Curve" <- w216
      n144 = Build Array(w201, w187, w190, w189) -> (w200:dbl[][])
      n145 = Build Array(w193, w192, w194, w196) -> (→"Accel_Result":dbl[])
      n146 = Bundle "Bundle"(w190, w189) -> (→"Aceel time vs Distance":cluster{dbl[], dbl[]})  [unwired: 1 in]
      n147 = Bundle "Bundle"(w190, w187) -> (→"Aceel time vs vehicle speed":cluster{dbl[], dbl[]})  [unwired: 1 in]
      n148 = Bundle "Bundle"(w187, w189) -> (→"vehicle speed vs Distance":cluster{dbl[], dbl[]})  [unwired: 1 in]
      n149 = Transpose 2D Array(2D array=w200) -> (transposed array=→"Vehicle_Total_Array":dbl[][])
      n150 = Build Array(w215, w214) -> (→"XY Graph 2":cluster{dbl[], dbl[]}[])
      n151 = Build Array(w218, w216) -> (→"XY Graph":cluster{"data":dbl[], "data":dbl[]}[])
    }
  }
